vi "Clear Errors.vi"(8 "error in (no error)":errorcluster, 11 "specific error code to clear (0: all)":i32[](array[numeric])) -> (0 "error out":errorcluster, 3 "specific error cleared?":bool)   [LabVIEW 2020, in "CSM-TagDisplayContainer.lvlib"]
uses:
  CSM-TagDisplayContainer.lvlib
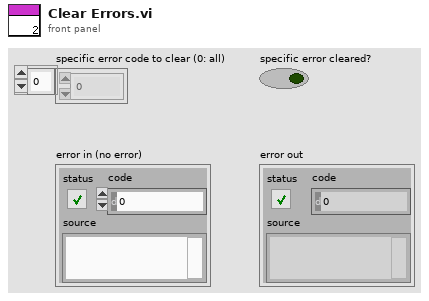
[diagram p1: front panel]
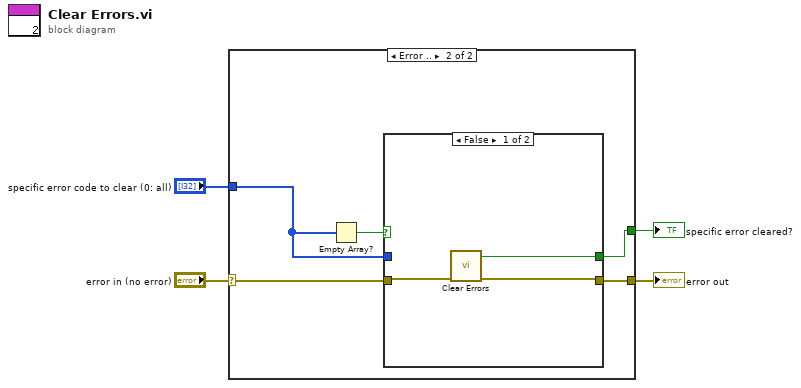
[diagram p0: block diagram]
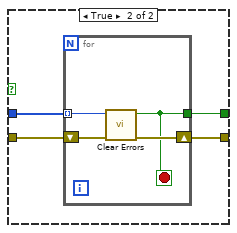
[diagram p3: hidden frame]
diagram:
  n1 = case shown="Error .." "error in (no error)" {
    selector: "error in (no error)" -> [w5 w8]
    tunnel: "specific error code to clear (0: all)" -> [_ w7]
    tunnel: [w5 w10] -> w3
    tunnel: [_ w9] -> w2
    frame No Error {
    }
    frame Error {
      n2 = Empty Array?(array=w7) -> (empty?=w6:bool)
      n3 = case shown="False" w6 {
        tunnel: [w12 w17] -> w10
        tunnel: [w11 w16] -> w9
        tunnel: w8 -> [w13 w15]
        tunnel: w7 -> [_ w14]
        frame False {
          n4 = call <vilib>:"Clear Errors.vi"("error in (no error)"=w13) -> ("error out"=w12:errorcluster, "specific error cleared?"=w11:bool)  [unwired: 5 in]
        }
        frame True {
          n5 = for {
            tunnel: w14 -> [w21] mode=indexing
            tunnel: [w18] -> w16
            shift-right: [w19] -> w17
            shift-left: w15 -> [w20]
            stop <- w18 stop-if-true
            n6 = call <vilib>:"Clear Errors.vi"("error in (no error)"=w20, "specific error code to clear (0: all)"=w21) -> ("error out"=w19:errorcluster, "specific error cleared?"=w18:bool)  [unwired: 4 in]
          }
        }
      }
    }
  }
  "error out" <- w3
  "specific error cleared?" <- w2
